vi "Update Cycle Count.vi"(8 "error in (no error)":errorcluster, 11 "Spectrum Recorder too in":refnum<class "Spectrum Recorder too.lvclass">) -> (0 "error out":errorcluster, 2 "Cycle count out":i32, 3 "Spectrum Recorder too out":refnum<class "Spectrum Recorder too.lvclass">)   [LabVIEW 2016, in "Spectrum Recorder too.lvclass"]
uses:
  Spectrum Recorder too.lvclass
  C:/github/Measure_core/Worker/Worker.lvclass
  Measure_core/Worker/Worker.lvclass/Worker.ctl
  NHMFL_Core/Libraries/Red Pitaya/RP Core/RP Transceiver/RP Transceiver.lvclass/RP Transceiver.ctl
  Measure_core/Worker/Read Cycle count.vi
  NHMFL_Core/Libraries/Red Pitaya/RP Core/RP Transceiver/Read Seen last phase word.vi
  NHMFL_Core/Libraries/Red Pitaya/RP Core/RP Transceiver/Write Seen last phase word.vi
  Measure_core/Worker/Write Cycle count.vi
  Read RP transceiver.vi
  Write RP transceiver.vi
  NHMFL_Core/Libraries/Red Pitaya/RP Core/RP Transceiver/RP Transceiver.lvclass
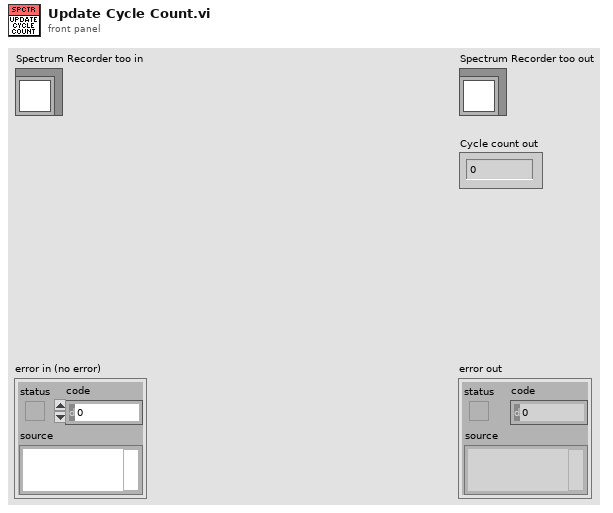
[diagram p1: front panel]
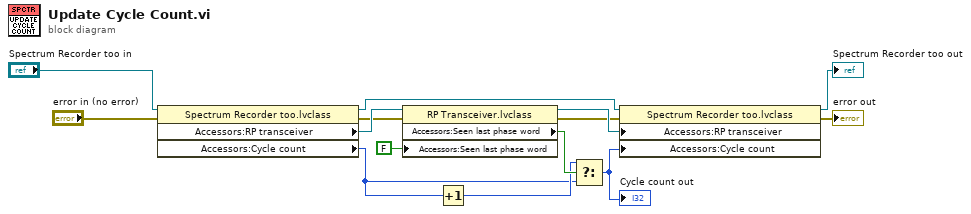
[diagram p0: block diagram]
diagram:
  n1 = property class="Spectrum Recorder too.lvclass"(reference="Spectrum Recorder too in", error in="error in (no error)") -> (reference out=w14:refnum<class "Spectrum Recorder too.lvclass">, error out=w7:errorcluster, "Accessors:RP transceiver"=w9:refnum<class "RP Transceiver.lvclass">, "Accessors:Cycle count"=w3:i32)
  n2 = property class="RP Transceiver.lvclass"(reference=w9, error in=w7, "Accessors:Seen last phase word"=FALSE ("Seen last phase word")) -> (reference out=w8:refnum<class "RP Transceiver.lvclass">, error out=w6:errorcluster, "Accessors:Seen last phase word"=w5:bool)
  n3 = Increment(x=w3) -> (x+1=w4:i32)
  n4 = Select(t=w4, s=w5, f=w3) -> (s? t:f=w2:i32)
  "Cycle count out" <- w2
  n5 = property class="Spectrum Recorder too.lvclass"(reference=w14, error in=w6, "Accessors:RP transceiver"=w8, "Accessors:Cycle count"=w2) -> (reference out=→"Spectrum Recorder too out":refnum<class "Spectrum Recorder too.lvclass">, error out=→"error out":errorcluster)
